vi "Paired_distances.vi"(8 "error in":errorcluster caption="entrée d'erreur", 9 "Y":string[][](array[string]), 10 "X":string[][](array[string]), 11 "paired_distances":cluster{"metric":string}={"metric"="euclidean"}) -> (0 "error out":errorcluster caption="sortie d'erreur", 3 "Data":T1)   [LabVIEW 2020]
doc: "Computes the paired distances between X and Y.\n\nComputes the distances between (X[0], Y[0]), (X[1], Y[1]), etc…\n\n\nParameters :\n\n- X : ndarray (n_samples, n_features)\nArray 1 for distance computation.\n\n- Y : ndarray (n_samples, n_features)\nArray 2 for distance computation.\n\n- metric : string or callable\nThe metric to use when calculating distance between instances in a feature array. If metric is a string, it must be one of the options specified in PAIRED_DISTANCES, including “euclidean”, “manhattan”, or “cosine”. Alternatively, if metric is a callable function, it is called on each pair of instances (rows) and the resulting value recorded. The callable should take two arrays from X as input and return a value indicating the distance between them.\n\nReturns :\n\n- distances : ndarray (n_samples, )"
uses:
  Paired_distances.lvclass
panel:
  out "Paired_distances.lvclass":refnum<class "Paired_distances.lvclass">
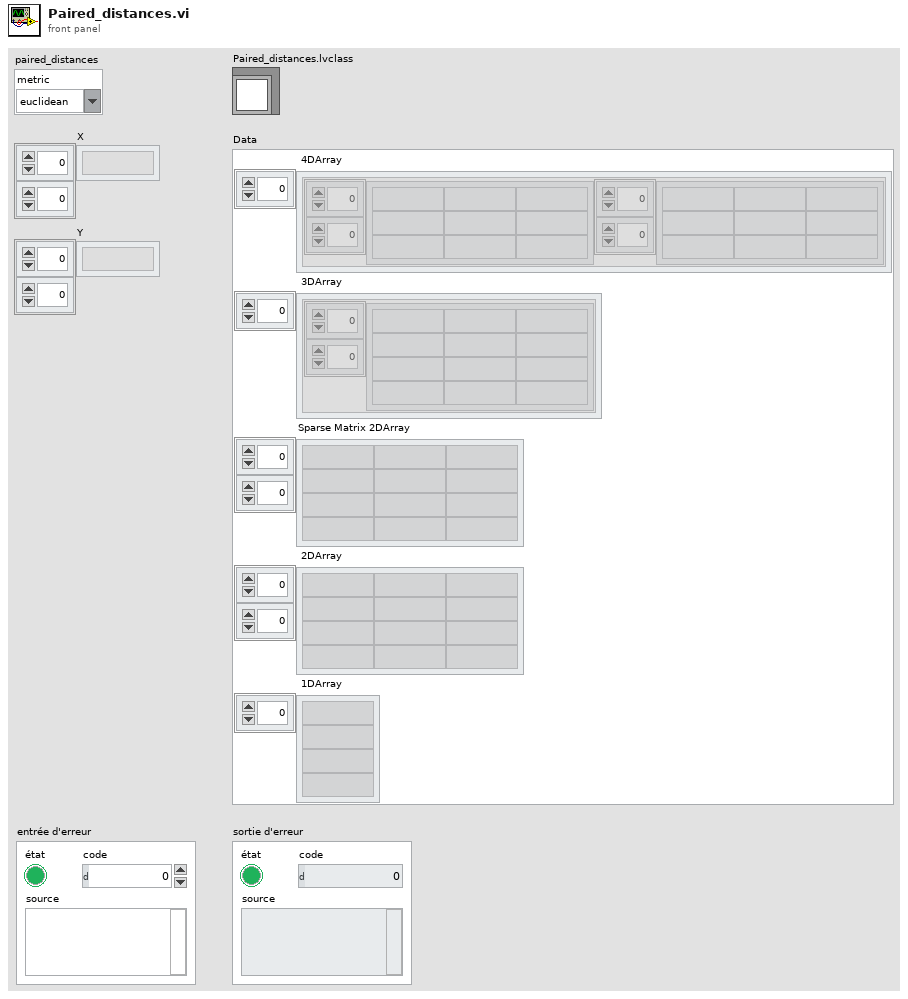
[diagram p1: front panel]
types:
  T1 = cluster{" 4DArray":cluster{"1":string[][], "2":string[][]}[], " 3DArray":cluster{"Tableau":string[][]}[], "Sparse Matrix 2DArray":string[][], " 2DArray":string[][], " 1DArray":string[]}
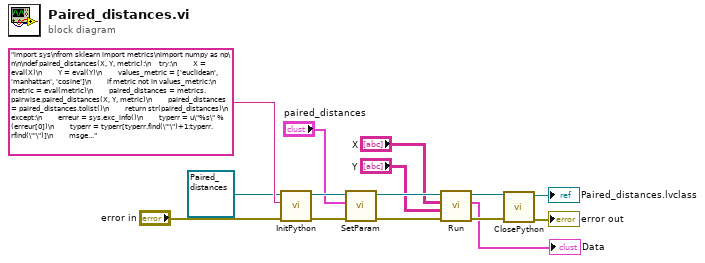
[diagram p0: block diagram]
diagram:
  n1 = call-dynamic "InitPython.vi"("error in (no error)"="error in", "Python Instruction"="import sys\nfrom sklearn import metrics\nimport numpy as np\n\n\ndef paired_distances(X, Y, metric):\n    try:\n        X = eval(X)\n        Y = eval(Y)\n        values_metric = ['euclidean', 'manhattan', 'cosine']\n        if metric not in values_metric:\n            metric = eval(metric)\n        paired_distances = metrics.pairwise.paired_distances(X, Y, metric)\n        paired_distances = paired_distances.tolist()\n        return str(paired_distances)\n    except:\n        erreur = sys.exc_info()\n        typerr = u\"%s\" % (erreur[0])\n        typerr = typerr[typerr.find(\"'\")+1:typerr.rfind(\"'\")]\n        msgerr = u\"%s\" % (erreur[1])\n        message = str('/!\\\\ {0} : {1}'. format(typerr,msgerr))\n        return message", "Scikit-learn en entrée"=refnum<class "Paired_distances.lvclass"> refnum ("Paired_distances.lvclass")) -> ("error out"=w10:errorcluster, "Scikit-learn en sortie"=w12:refnum<class "Paired_distances.lvclass">)  [unwired: 7 in]
  n2 = call-dynamic "SetParam.vi"("error in (no error)"=w10, "paired_distances"="paired_distances", "Paired_distances.lvclass"=w12) -> ("error out"=w8:errorcluster, "Paired_distances.lvclass"=w9:refnum<class "Paired_distances.lvclass">)  [unwired: 7 in]
  n3 = call-dynamic "Run.vi"("error in (no error)"=w8, "Y"="Y", "X"="X", "Paired_distances.lvclass"=w9) -> ("error out"=w6:errorcluster, "Data"=→"Data":T1, "Paired_distances.lvclass"=w7:refnum<class "Paired_distances.lvclass">)  [unwired: 5 in]
  n4 = call-dynamic "ClosePython.vi"("error in (no error)"=w6, "Scikit-learn en entrée"=w7) -> ("error out"=→"error out":errorcluster, "Scikit-learn en sortie"=→"Paired_distances.lvclass":refnum<class "Paired_distances.lvclass">)  [unwired: 8 in]
